vi "Rear IO Panel.vi"(11 "Full System Configuration":T2={"Rack"=enum."15U; 1-Phase; 16A; 100-240V", "Middle Rail"=enum."None", "Ballast"={"Main"=0, "Small"=0, "Side"=0}, "Front Panel I/O"={"EMO Button"=FALSE, "USB 3.0"=FALSE, "Display"=FALSE, "1st USB 2.0"=FALSE, "2nd USB 2.0"=FALSE, "Ethernet 3"=FALSE, "EMO Extension (3rd Party)"=FALSE, "EMO Extension (Rack In & Out)"=FALSE, "Aux Dual C13 QAC Outlets"=FALSE, "Residual-current Circuit Breaker"=FALSE, "Serial"=FALSE, "GPIB"=FALSE}, "Rear Panel I/O"={"Rear Panel I/O Configuration"=enum."Blank Panel", "EMO Button"=FALSE, "Power, Status & Banana Ground"=FALSE, "Ethernet 2"=FALSE, "Display"=FALSE, "USB 3.0"=FALSE, "DIO"=FALSE, "GPIB"=FALSE, "Aux Dual C13 QAC Outlets"=FALSE, "Residual-current Circuit Breaker"=FALSE, "Serial"=FALSE, "SMA"=FALSE}, "Miscellaneous Options"={"Eyebolts"=FALSE, "Tower Light"=FALSE, "Top/Side Monitor Mount Kit"=FALSE, "24\" Monitor"=FALSE, "Keyboard & Mouse"=FALSE, "Secondary Ethernet Switch"=FALSE, "Extra USB Hub"=FALSE, "USB-6509"=FALSE, "Front Door"=enum."38U (Solid) IG", "Primary Ethernet Switch"=enum."Item 0", "Use Posture"=enum."Item 0"}, "Accessories"={"Screw Type"=enum."10-32", "Cage Nuts & Screws"=0.0, "Filler Panel Color"=enum."Interface Gray", "1U"=0.0, "2U"=0.0, "3U"=0.0}} {"Ballast"."Side" max=5 step=1; "Ballast"."Small" max=5 step=1; "Ballast"."Main" max=5 step=1}) -> (3 "Array":T1[](array[typedef]))   [LabVIEW 2023]
uses:
  Option Type Defs/Full System Configuration.ctl
  Option Type Defs/Rack.ctl
  Option Type Defs/Middle Rail.ctl
  Option Type Defs/Ballast.ctl
  Option Type Defs/Front Panel IO.ctl
  Option Type Defs/Rear Panel IO.ctl
  Option Type Defs/Rear Panel IO Configuration.ctl
  Option Type Defs/Miscellaneous Options.ctl
  Option Type Defs/Front Door.ctl
  Option Type Defs/Accessories.ctl
  Option Type Defs/Screw Types.ctl
  Option Type Defs/Filler Panel Color.ctl
  Option Type Defs/Parts List.ctl
  <userlib>/_OpenG.lib/lvdata/lvdata.llb/openg_variant.lvlib
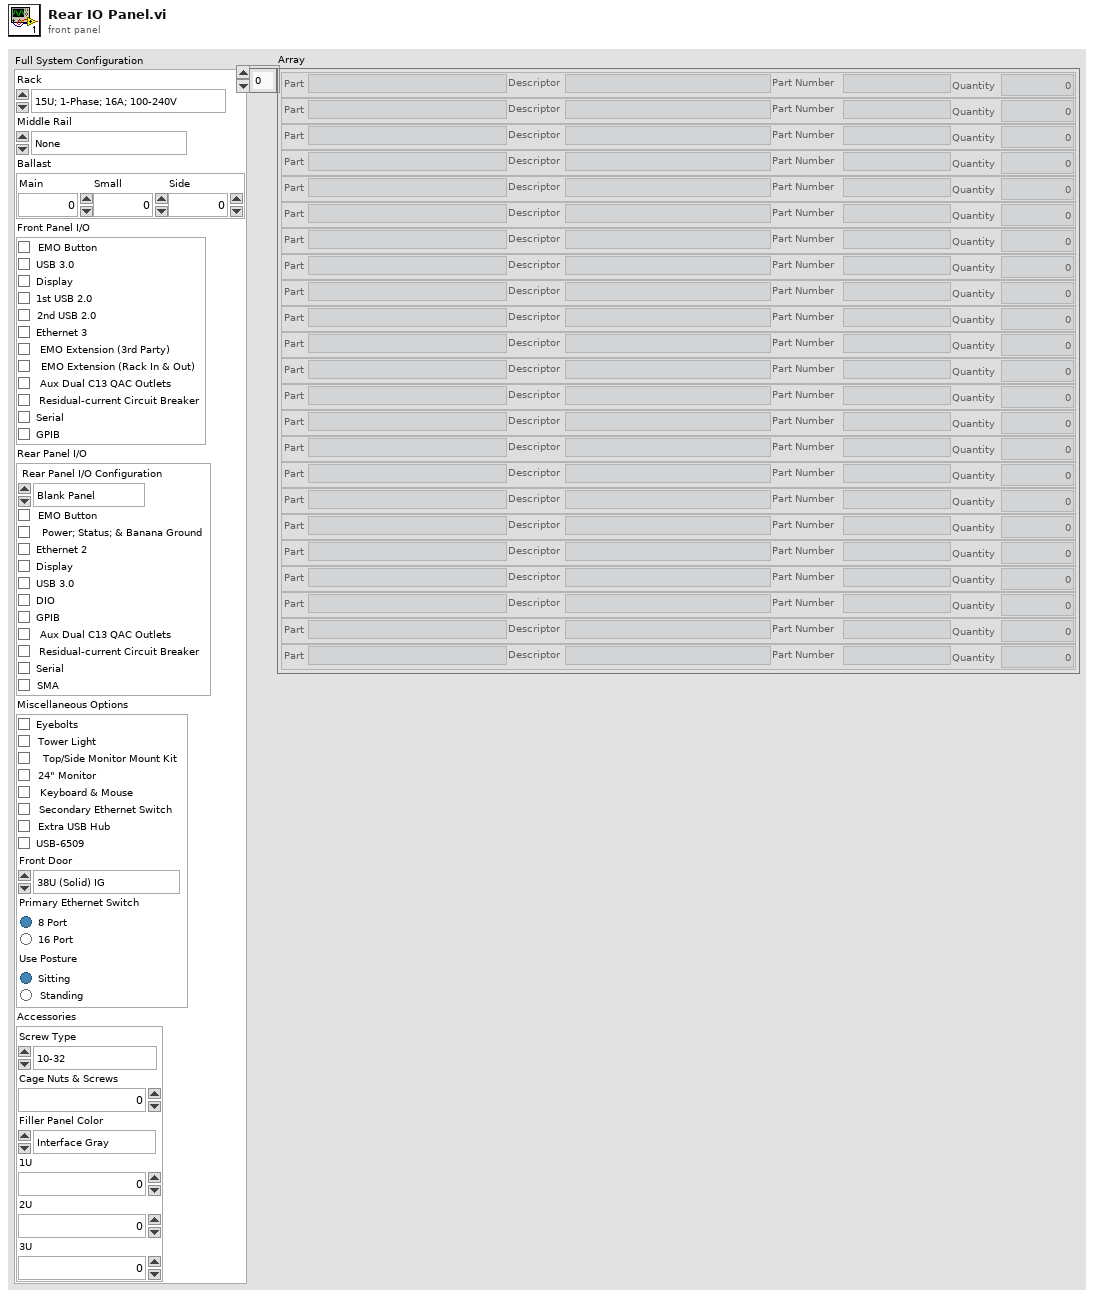
[diagram p1: front panel]
types:
  T1 = typedef "Parts List.ctl" = cluster{"Part":string, "Descriptor":string, "Part Number":string, "Quantity":dbl}
  T2 = typedef "Full System Configuration.ctl" = cluster{"Rack":T3, "Middle Rail":T4, "Ballast":T5, "Front Panel I/O":T6, "Rear Panel I/O":T7, "Miscellaneous Options":T9, "Accessories":T11}
  T3 = typedef "Rack.ctl" = enum16{"15U; 1-Phase; 16A; 100-240V", "15U; 1-Phase; 24A; 100-240V", "38U; 3-Phase Delta; 50A; 200-240V", "38U; 1-Phase; 24A; 100-120V", "38U; 3-Phase Wye; 50A; 200-240V", "38U; 3-Phase Delta; 50A; 380-480V", "38U; 3-Phase Delta; 32A; 200-240V", "38U; 3-Phase Wye; 16A; 100-240V", "44U; 1-Phase; 24A; 100-240V", "44U; 3-Phase Delta; 32A; 200-240V"}
  T4 = typedef "Middle Rail.ctl" = enum16{"None", "Flip Side Rear; D=168.83mm", "Parallel Rear; D=145mm", "Flip Side Front; D=145mm", "Parallel Front; D=145mm"}
  T5 = typedef "Ballast.ctl" = cluster{"Main":u16, "Small":u16, "Side":u16}
  T6 = typedef "Front Panel IO.ctl" = cluster{"EMO Button":bool, "USB 3.0":bool, "Display":bool, "1st USB 2.0":bool, "2nd USB 2.0":bool, "Ethernet 3":bool, "EMO Extension (3rd Party)":bool, "EMO Extension (Rack In & Out)":bool, "Aux Dual C13 QAC Outlets":bool, "Residual-current Circuit Breaker":bool, "Serial":bool, "GPIB":bool}
  T7 = typedef "Rear Panel IO.ctl" = cluster{"Rear Panel I/O Configuration":T8, "EMO Button":bool, "Power, Status & Banana Ground":bool, "Ethernet 2":bool, "Display":bool, "USB 3.0":bool, "DIO":bool, "GPIB":bool, "Aux Dual C13 QAC Outlets":bool, "Residual-current Circuit Breaker":bool, "Serial":bool, "SMA":bool}
  T8 = typedef "Rear Panel IO Configuration.ctl" = enum16{"Blank Panel", "Fully Populated Panel", "Custom Panel"}
  T9 = typedef "Miscellaneous Options.ctl" = cluster{"Eyebolts":bool, "Tower Light":bool, "Top/Side Monitor Mount Kit":bool, "24\" Monitor":bool, "Keyboard & Mouse":bool, "Secondary Ethernet Switch":bool, "Extra USB Hub":bool, "USB-6509":bool, "Front Door":T10, "Primary Ethernet Switch":enum32{"Item 0", "Item 1"}, "Use Posture":enum32{"Item 0", "Item 1"}}
  T10 = typedef "Front Door.ctl" = enum16{"None", "38U (Solid) IG", "38U (Solid) EG", "38U: Top 14U (Solid) IG", "38U (Clear) IG", "44U (Solid) IG", "44U (Solid) EG"}
  T11 = typedef "Accessories.ctl" = cluster{"Screw Type":T12, "Cage Nuts & Screws":dbl, "Filler Panel Color":T13, "1U":dbl, "2U":dbl, "3U":dbl}
  T12 = typedef "Screw Types.ctl" = enum16{"None", "M6 (Most Common)", "10-32", "12-24"}
  T13 = typedef "Filler Panel Color.ctl" = enum16{"None", "Interface Gray", "Environmental Gray"}
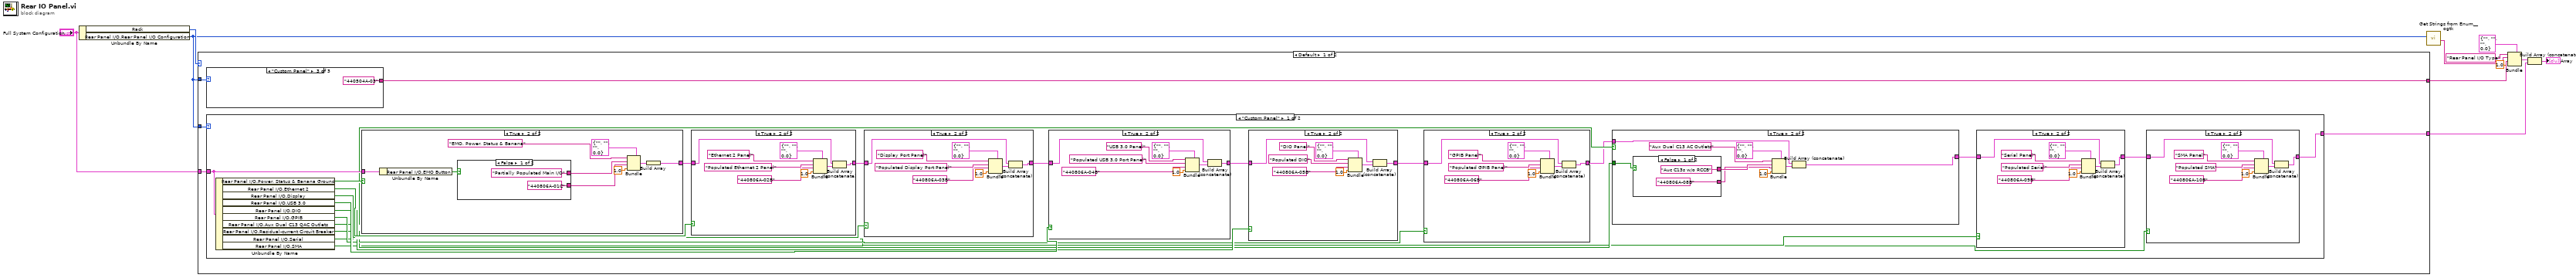
[diagram p0: block diagram]
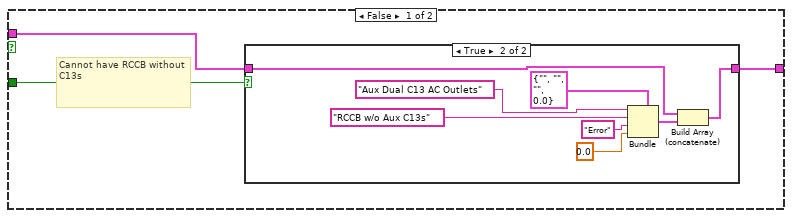
[diagram p4: hidden frame]
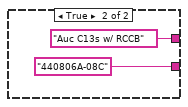
[diagram p6: hidden frame]
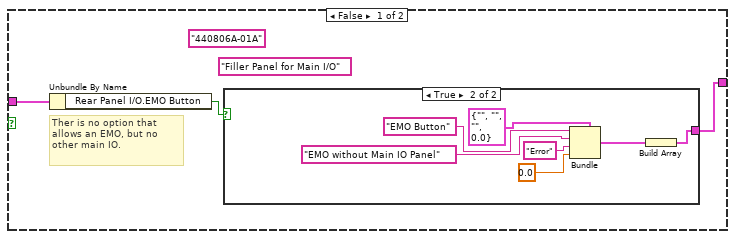
[diagram p12: hidden frame]
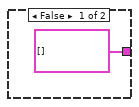
[diagram p13: hidden frame]
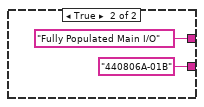
[diagram p14: hidden frame]
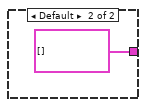
[diagram p15: hidden frame]
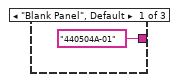
[diagram p16: hidden frame]
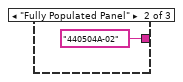
[diagram p17: hidden frame]
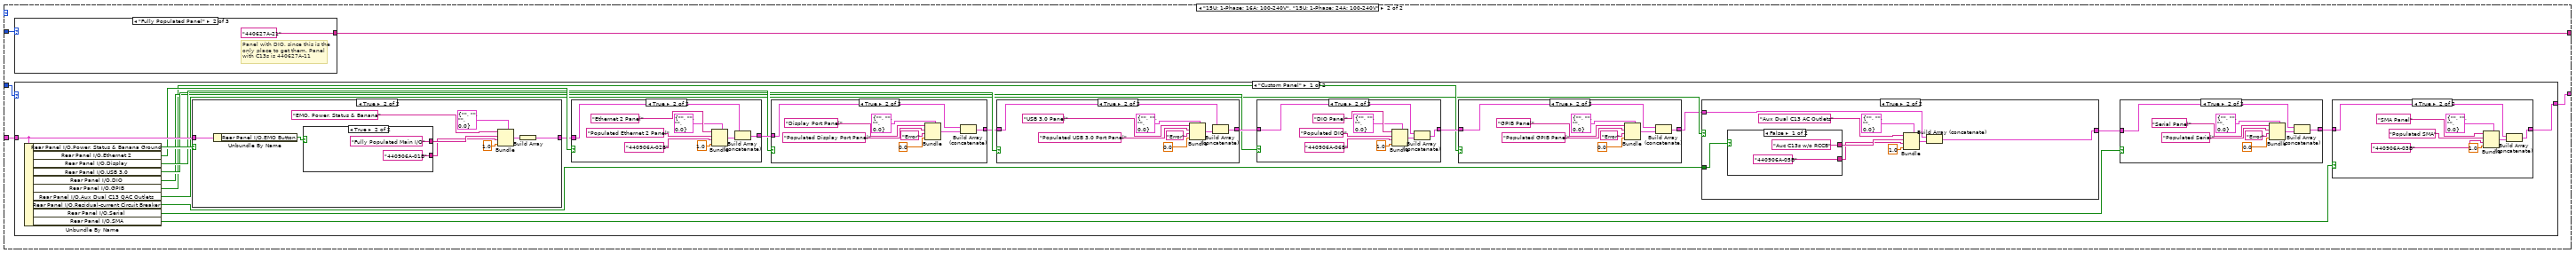
[diagram p18: hidden frame]
diagram:
  n1 = Unbundle By Name("Full System Configuration") -> ("Rack"=w5:T3, "Rear Panel I/O.Rear Panel I/O Configuration"=w4:T8)
  n2 = case shown="Default" w5 {
    tunnel: w4 -> [w16 w157]
    tunnel: [w15 w156] -> w9
    tunnel: w4 -> [w14 w155]
    tunnel: "Full System Configuration" -> [w13 w154]
    tunnel: [w12 w153] -> w2
    frame Default {
      n3 = case shown="\"Custom Panel\"" w16 {
        tunnel: ["440504A-01" "440504A-02" "440504A-03"] -> w15
        frame "Blank Panel", Default {
        }
        frame "Fully Populated Panel" {
        }
        frame "Custom Panel" {
        }
      }
      n4 = case shown="\"Custom Panel\"" w14 {
        tunnel: w13 -> [w35 _]
        tunnel: [w19 T1[] []] -> w12
        frame "Custom Panel" {
          n5 = Unbundle By Name(w35) -> ("Rear Panel I/O.Power, Status & Banana Ground"=w36:bool, "Rear Panel I/O.Ethernet 2"=w34:bool, "Rear Panel I/O.Display"=w31:bool, "Rear Panel I/O.USB 3.0"=w28:bool, "Rear Panel I/O.DIO"=w26:bool, "Rear Panel I/O.GPIB"=w25:bool, "Rear Panel I/O.Aux Dual C13 QAC Outlets"=w24:bool, "Rear Panel I/O.Residual-current Circuit Breaker"=w23:bool, "Rear Panel I/O.Serial"=w18:bool, "Rear Panel I/O.SMA"=w17:bool)
          n6 = case shown="True" w36 {
            tunnel: w35 -> [w127 w144]
            tunnel: [w125 w137] -> w33
            frame False {
              (unwired) "440806A-01A" ("Part Number")
              (unwired) "Filler Panel for Main I/O"
              # "Ther is no option that allows an EMO, but no other main IO."
              n7 = Unbundle By Name(w127) -> ("Rear Panel I/O.EMO Button"=w126:bool)
              n8 = case shown="True" w126 {
                tunnel: [T1[] [] w130] -> w125
                frame False {
                }
                frame True {
                  n9 = Bundle(cluster=T1 {"Part"="", "Descriptor"="", "Part Number"="", "Quantity"=0.0}, "Part"="EMO Button", "Descriptor"="EMO without Main IO Panel", "Part Number"="Error", "Quantity"=0.0) -> (w131:T1)
                  n10 = Build Array(w131) -> (w130:T1[])
                }
              }
            }
            frame True {
              n11 = Unbundle By Name(w144) -> ("Rear Panel I/O.EMO Button"=w143:bool)
              n12 = case shown="False" w143 {
                tunnel: ["Partially Populated Main I/O" "Fully Populated Main I/O"] -> w140
                tunnel: ["440806A-01C" ("Part Number") "440806A-01B" ("Part Number")] -> w139
                frame False {
                }
                frame True {
                }
              }
              n13 = Bundle(cluster=T1 {"Part"="", "Descriptor"="", "Part Number"="", "Quantity"=0.0}, "Part"="EMO, Power, Status & Banana", "Descriptor"=w140, "Part Number"=w139, "Quantity"=1.0) -> (w138:T1)
              n14 = Build Array(w138) -> (w137:T1[])
            }
          }
          n15 = case shown="True" w34 {
            tunnel: w33 -> [w116 w124]
            tunnel: [w116 w118] -> w32
            frame False {
            }
            frame True {
              n16 = Bundle(cluster=T1 {"Part"="", "Descriptor"="", "Part Number"="", "Quantity"=0.0}, "Part"="Ethernet 2 Panel", "Descriptor"="Populated Ethernet 2 Panel", "Part Number"="440806A-02B", "Quantity"=1.0) -> (w119:T1)
              n17 = Build Array (concatenate)(w124, w119) -> (w118:T1[])
            }
          }
          n18 = case shown="True" w31 {
            tunnel: w32 -> [w107 w115]
            tunnel: [w107 w109] -> w27
            frame False {
            }
            frame True {
              n19 = Bundle(cluster=T1 {"Part"="", "Descriptor"="", "Part Number"="", "Quantity"=0.0}, "Part"="Display Port Panel", "Descriptor"="Populated Display Port Panel", "Part Number"="440806A-03B", "Quantity"=1.0) -> (w110:T1)
              n20 = Build Array (concatenate)(w115, w110) -> (w109:T1[])
            }
          }
          n21 = case shown="True" w28 {
            tunnel: w27 -> [w98 w106]
            tunnel: [w98 w100] -> w30
            frame False {
            }
            frame True {
              n22 = Bundle(cluster=T1 {"Part"="", "Descriptor"="", "Part Number"="", "Quantity"=0.0}, "Part"="USB 3.0 Panel", "Descriptor"="Populated USB 3.0 Port Panel", "Part Number"="440806A-04B", "Quantity"=1.0) -> (w101:T1)
              n23 = Build Array (concatenate)(w106, w101) -> (w100:T1[])
            }
          }
          n24 = case shown="True" w26 {
            tunnel: w30 -> [w89 w97]
            tunnel: [w89 w91] -> w29
            frame False {
            }
            frame True {
              n25 = Bundle(cluster=T1 {"Part"="", "Descriptor"="", "Part Number"="", "Quantity"=0.0}, "Part"="DIO Panel", "Descriptor"="Populated DIO", "Part Number"="440806A-05B", "Quantity"=1.0) -> (w92:T1)
              n26 = Build Array (concatenate)(w97, w92) -> (w91:T1[])
            }
          }
          n27 = case shown="True" w25 {
            tunnel: w29 -> [w80 w88]
            tunnel: [w80 w82] -> w22
            frame False {
            }
            frame True {
              n28 = Bundle(cluster=T1 {"Part"="", "Descriptor"="", "Part Number"="", "Quantity"=0.0}, "Part"="GPIB Panel", "Descriptor"="Populated GPIB Panel", "Part Number"="440806A-06B", "Quantity"=1.0) -> (w83:T1)
              n29 = Build Array (concatenate)(w88, w83) -> (w82:T1[])
            }
          }
          n30 = case shown="True" w24 {
            tunnel: [w57 w70] -> w21
            tunnel: w23 -> [w56 w69]
            tunnel: w22 -> [w55 w68]
            frame False {
              # "Cannot have RCCB without C13s"
              n31 = case shown="True" w56 {
                tunnel: [w58 w61] -> w57
                tunnel: w55 -> [w58 w60]
                frame False {
                }
                frame True {
                  n32 = Bundle(cluster=T1 {"Part"="", "Descriptor"="", "Part Number"="", "Quantity"=0.0}, "Part"="Aux Dual C13 AC Outlets", "Descriptor"="RCCB w/o Aux C13s", "Part Number"="Error", "Quantity"=0.0) -> (w62:T1)
                  n33 = Build Array (concatenate)(w60, w62) -> (w61:T1[])
                }
              }
            }
            frame True {
              n34 = case shown="False" w69 {
                tunnel: ["Auc C13s w/o RCCB" "Auc C13s w/ RCCB"] -> w73
                tunnel: ["440806A-08B" ("Part Number") "440806A-08C" ("Part Number")] -> w72
                frame False {
                }
                frame True {
                }
              }
              n35 = Bundle(cluster=T1 {"Part"="", "Descriptor"="", "Part Number"="", "Quantity"=0.0}, "Part"="Aux Dual C13 AC Outlets", "Descriptor"=w73, "Part Number"=w72, "Quantity"=1.0) -> (w71:T1)
              n36 = Build Array (concatenate)(w68, w71) -> (w70:T1[])
            }
          }
          n37 = case shown="True" w18 {
            tunnel: w21 -> [w46 w54]
            tunnel: [w46 w48] -> w20
            frame False {
            }
            frame True {
              n38 = Bundle(cluster=T1 {"Part"="", "Descriptor"="", "Part Number"="", "Quantity"=0.0}, "Part"="Serial Panel", "Descriptor"="Populated Serial", "Part Number"="440806A-09B", "Quantity"=1.0) -> (w49:T1)
              n39 = Build Array (concatenate)(w54, w49) -> (w48:T1[])
            }
          }
          n40 = case shown="True" w17 {
            tunnel: w20 -> [w37 w45]
            tunnel: [w37 w39] -> w19
            frame False {
            }
            frame True {
              n41 = Bundle(cluster=T1 {"Part"="", "Descriptor"="", "Part Number"="", "Quantity"=0.0}, "Part"="SMA Panel", "Descriptor"="Populated SMA", "Part Number"="440806A-10B", "Quantity"=1.0) -> (w40:T1)
              n42 = Build Array (concatenate)(w45, w40) -> (w39:T1[])
            }
          }
        }
        frame Default {
        }
      }
    }
    frame "15U; 1-Phase; 16A; 100-240V", "15U; 1-Phase; 24A; 100-240V" {
      n43 = case shown="\"Fully Populated Panel\"" w157 {
        tunnel: ["440627A-01" "440627A-21" "440627A-12"] -> w156
        frame "Blank Panel", Default {
        }
        frame "Fully Populated Panel" {
          # "Panel with DIO, since this is the only place to get them. Panel with C13s is 440627A-11"
        }
        frame "Custom Panel" {
        }
      }
      n44 = case shown="\"Custom Panel\"" w155 {
        tunnel: w154 -> [w176 _]
        tunnel: [w160 T1[] []] -> w153
        frame "Custom Panel" {
          n45 = Unbundle By Name(w176) -> ("Rear Panel I/O.Power, Status & Banana Ground"=w177:bool, "Rear Panel I/O.Ethernet 2"=w175:bool, "Rear Panel I/O.Display"=w172:bool, "Rear Panel I/O.USB 3.0"=w169:bool, "Rear Panel I/O.DIO"=w167:bool, "Rear Panel I/O.GPIB"=w166:bool, "Rear Panel I/O.Aux Dual C13 QAC Outlets"=w165:bool, "Rear Panel I/O.Residual-current Circuit Breaker"=w164:bool, "Rear Panel I/O.Serial"=w159:bool, "Rear Panel I/O.SMA"=w158:bool)
          n46 = case shown="True" w177 {
            tunnel: w176 -> [w268 w284]
            tunnel: [w266 w277] -> w174
            frame False {
              (unwired) "440806A-01A" ("Part Number")
              (unwired) "Filler Panel for Main I/O"
              # "Ther is no option that allows an EMO, but no other main IO."
              n47 = Unbundle By Name(w268) -> ("Rear Panel I/O.EMO Button"=w267:bool)
              n48 = case shown="False" w267 {
                tunnel: [T1[] [] w270] -> w266
                frame False {
                }
                frame True {
                  n49 = Bundle(cluster=T1 {"Part"="", "Descriptor"="", "Part Number"="", "Quantity"=0.0}, "Part"="EMO Button", "Descriptor"="EMO without Main IO Panel", "Part Number"="Error") -> (w271:T1)  [unwired: 1 in]
                  n50 = Build Array(w271) -> (w270:T1[])
                }
              }
            }
            frame True {
              n51 = Unbundle By Name(w284) -> ("Rear Panel I/O.EMO Button"=w283:bool)
              n52 = case shown="True" w283 {
                tunnel: ["Partially Populated Main I/O" "Fully Populated Main I/O"] -> w280
                tunnel: ["440906A-01C" ("Part Number") "440906A-01B" ("Part Number")] -> w279
                frame False {
                }
                frame True {
                }
              }
              n53 = Bundle(cluster=T1 {"Part"="", "Descriptor"="", "Part Number"="", "Quantity"=0.0}, "Part"="EMO, Power, Status & Banana", "Descriptor"=w280, "Part Number"=w279, "Quantity"=1.0) -> (w278:T1)
              n54 = Build Array(w278) -> (w277:T1[])
            }
          }
          n55 = case shown="True" w175 {
            tunnel: w174 -> [w257 w265]
            tunnel: [w257 w259] -> w173
            frame False {
            }
            frame True {
              n56 = Bundle(cluster=T1 {"Part"="", "Descriptor"="", "Part Number"="", "Quantity"=0.0}, "Part"="Ethernet 2 Panel", "Descriptor"="Populated Ethernet 2 Panel", "Part Number"="440906A-02B", "Quantity"=1.0) -> (w260:T1)
              n57 = Build Array (concatenate)(w265, w260) -> (w259:T1[])
            }
          }
          n58 = case shown="True" w172 {
            tunnel: w173 -> [w248 w256]
            tunnel: [w248 w250] -> w168
            frame False {
            }
            frame True {
              n59 = Bundle(cluster=T1 {"Part"="", "Descriptor"="", "Part Number"="", "Quantity"=0.0}, "Part"="Display Port Panel", "Descriptor"="Populated Display Port Panel", "Part Number"="Error", "Quantity"=0.0) -> (w251:T1)
              n60 = Build Array (concatenate)(w256, w251) -> (w250:T1[])
            }
          }
          n61 = case shown="True" w169 {
            tunnel: w168 -> [w239 w247]
            tunnel: [w239 w241] -> w171
            frame False {
            }
            frame True {
              n62 = Bundle(cluster=T1 {"Part"="", "Descriptor"="", "Part Number"="", "Quantity"=0.0}, "Part"="USB 3.0 Panel", "Descriptor"="Populated USB 3.0 Port Panel", "Part Number"="Error", "Quantity"=0.0) -> (w242:T1)
              n63 = Build Array (concatenate)(w247, w242) -> (w241:T1[])
            }
          }
          n64 = case shown="True" w167 {
            tunnel: w171 -> [w230 w238]
            tunnel: [w230 w232] -> w170
            frame False {
            }
            frame True {
              n65 = Bundle(cluster=T1 {"Part"="", "Descriptor"="", "Part Number"="", "Quantity"=0.0}, "Part"="DIO Panel", "Descriptor"="Populated DIO", "Part Number"="440906A-06B", "Quantity"=1.0) -> (w233:T1)
              n66 = Build Array (concatenate)(w238, w233) -> (w232:T1[])
            }
          }
          n67 = case shown="True" w166 {
            tunnel: w170 -> [w221 w229]
            tunnel: [w221 w223] -> w163
            frame False {
            }
            frame True {
              n68 = Bundle(cluster=T1 {"Part"="", "Descriptor"="", "Part Number"="", "Quantity"=0.0}, "Part"="GPIB Panel", "Descriptor"="Populated GPIB Panel", "Part Number"="Error", "Quantity"=0.0) -> (w224:T1)
              n69 = Build Array (concatenate)(w229, w224) -> (w223:T1[])
            }
          }
          n70 = case shown="True" w165 {
            tunnel: [w198 w211] -> w162
            tunnel: w164 -> [w197 w210]
            tunnel: w163 -> [w196 w209]
            frame False {
              # "Cannot have RCCB without C13s"
              n71 = case shown="False" w197 {
                tunnel: [w199 w202] -> w198
                tunnel: w196 -> [w199 w201]
                frame False {
                }
                frame True {
                  n72 = Bundle(cluster=T1 {"Part"="", "Descriptor"="", "Part Number"="", "Quantity"=0.0}, "Part"="Aux Dual C13 AC Outlets", "Descriptor"="RCCB w/o Aux C13s", "Part Number"="Error", "Quantity"=0.0) -> (w203:T1)
                  n73 = Build Array (concatenate)(w201, w203) -> (w202:T1[])
                }
              }
            }
            frame True {
              n74 = case shown="False" w210 {
                tunnel: ["Auc C13s w/o RCCB" "Auc C13s w/ RCCB"] -> w214
                tunnel: ["440906A-05B" ("Part Number") "440906A-05C" ("Part Number")] -> w213
                frame False {
                }
                frame True {
                }
              }
              n75 = Bundle(cluster=T1 {"Part"="", "Descriptor"="", "Part Number"="", "Quantity"=0.0}, "Part"="Aux Dual C13 AC Outlets", "Descriptor"=w214, "Part Number"=w213, "Quantity"=1.0) -> (w212:T1)
              n76 = Build Array (concatenate)(w209, w212) -> (w211:T1[])
            }
          }
          n77 = case shown="True" w159 {
            tunnel: w162 -> [w187 w195]
            tunnel: [w187 w189] -> w161
            frame False {
            }
            frame True {
              n78 = Bundle(cluster=T1 {"Part"="", "Descriptor"="", "Part Number"="", "Quantity"=0.0}, "Part"="Serial Panel", "Descriptor"="Populated Serial", "Part Number"="Error", "Quantity"=0.0) -> (w190:T1)
              n79 = Build Array (concatenate)(w195, w190) -> (w189:T1[])
            }
          }
          n80 = case shown="True" w158 {
            tunnel: w161 -> [w178 w186]
            tunnel: [w178 w180] -> w160
            frame False {
            }
            frame True {
              n81 = Bundle(cluster=T1 {"Part"="", "Descriptor"="", "Part Number"="", "Quantity"=0.0}, "Part"="SMA Panel", "Descriptor"="Populated SMA", "Part Number"="440906A-03B", "Quantity"=1.0) -> (w181:T1)
              n82 = Build Array (concatenate)(w186, w181) -> (w180:T1[])
            }
          }
        }
        frame Default {
        }
      }
    }
  }
  n83 = call <userlib>:"Get Strings from Enum__ogtk.vi"("Enum"=w4) -> ("String Value"=w8:string)  [unwired: 7 in, 3 out]
  n84 = Bundle(cluster=T1 {"Part"="", "Descriptor"="", "Part Number"="", "Quantity"=0.0}, "Part"="Rear Panel I/O Type", "Descriptor"=w8, "Part Number"=w9, "Quantity"=1.0) -> (w10:T1)
  n85 = Build Array (concatenate)(w10, w2) -> (→"Array":T1[])
